vi "record data in array.vi"(2 "clear data":bool, 3 "input data":u8) -> (0 "data array length":u8, 1 "recorded data array":u8[](array[numeric]))   [LabVIEW 2009]
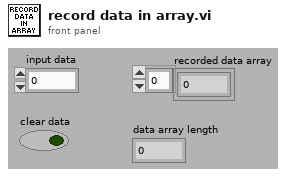
[diagram p1: front panel]
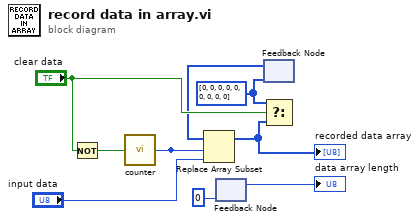
[diagram p0: block diagram]
diagram:
  w6 = u8[] [0, 0, 0, 0, 0, 0, 0, 0, 0]
  n1 = Not(x="clear data") -> (.not. x?=w10:bool)
  n2 = call "counter.vi"("reset"=w10) -> ("count"=w3:u8)
  n3 = feedback #1(u8 0 ("count")) -> (→"data array length":u8)
  n4 = feedback #2(w6) -> (w2:u8[])
  n5 = Replace Array Subset(array=w2, new element="input data", index=w3) -> (w9:u8[])
  "recorded data array" <- w9
  n6 = Select(t=w6, s="clear data", f=w9) -> (s? t:f=w7:u8[])
